vi "Multiplication.vi"() -> ()   [LabVIEW 2022 SP3]
panel:
  out "X":dbl
  in  "B":dbl
  in  "A":dbl
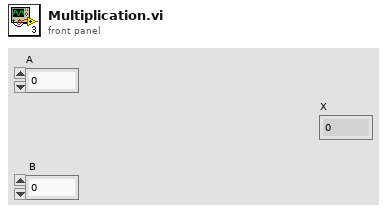
[diagram p1: front panel]
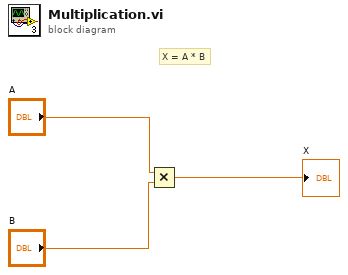
[diagram p0: block diagram]
diagram:
  # "X = A * B"
  n1 = Multiply(x="A", y="B") -> (x*y=→"X":dbl)
